vi "container.vi"   [LabVIEW 2014]
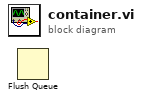
[diagram p0: block diagram]
diagram:
  n1 = Flush Queue() -> ()  [unwired: 2 in, 3 out]
